vi "FPGA_AIWriteAccumulatorCenter.vi"(8 "error in (no error)":errorcluster, 9 "Center":i32, 10 "Channel":T1=enum."AI 1", 11 "AI Reference in":T2) -> (0 "error out":errorcluster, 3 "AI Reference out":T2)   [LabVIEW 2017]
uses:
  <vilib>/Rock Robotics/SystemInterfaces/AI/FPGA_AIDevRef.ctl
  <vilib>/Rock Robotics/SystemInterfaces/AI/FPGA_AIChannel.ctl
  <vilib>/Rock Robotics/SystemInterfaces/System/FPGA_SystemFPGA Ref Global.vi
  <vilib>/Utility/error.llb/Error Cluster From Error Code.vi
  <vilib>/rvi/errors/niLvFpgaAdjustHostInterfaceError.vi
  <vilib>/rvi/interface/nirviReadWriteControl/nirviReadWriteControl.xnode
  <vilib>/Rock Robotics/SystemInterfaces/System/FPGA_SystemFRC FPGA Ref.ctl
  <vilib>/rvi/interface/Simulation/niFpgaSimulationCallBeginRW.vi
  NiFpgaLv.dll
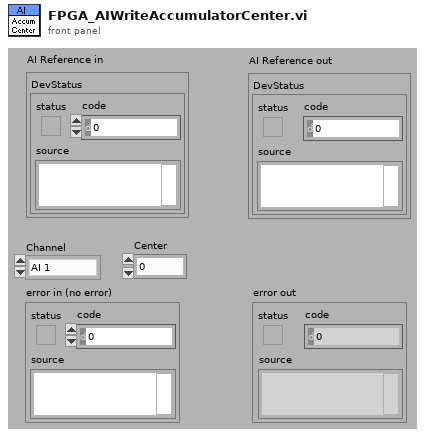
[diagram p1: front panel]
types:
  T1 = typedef "FPGA_AIChannel.ctl" = enum8{"AI 0", "AI 1", "AI 2", "AI 3", "AI MXP 0", "AI MXP 1", "AI MXP 2", "AI MXP 3", "Invalid"}
  T2 = typedef "FPGA_AIDevRef.ctl" = cluster{"DevStatus":errorcluster}
  T3 = typedef "FPGA_SystemFRC FPGA Ref.ctl" = refnum<k20>
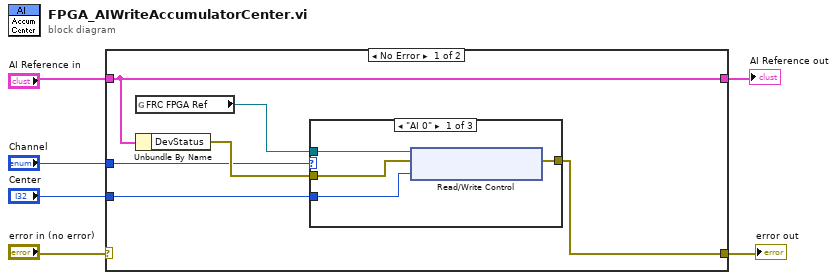
[diagram p0: block diagram]
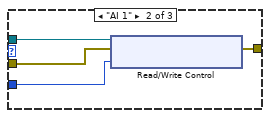
[diagram p2: hidden frame]
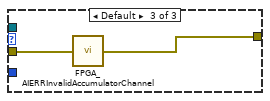
[diagram p3: hidden frame]
diagram:
  n1 = case shown="No Error" "error in (no error)" {
    selector: "error in (no error)" -> [_ w23]
    tunnel: [w12 w24] -> w5
    tunnel: "AI Reference in" -> [w12 w24]
    tunnel: [w9 w23] -> w3
    tunnel: "Center" -> [w10 _]
    tunnel: "Channel" -> [w8 _]
    frame No Error {
      n2 = global read "FPGA_SystemFPGA Ref Global.vi" "FRC FPGA Ref"() -> (w7:T3)
      n3 = Unbundle By Name(w12) -> ("DevStatus"=w11:errorcluster)
      n4 = case shown="\"AI 0\"" w8 {
        tunnel: w11 -> [w14 w18 w22]
        tunnel: [w16 w19 w21] -> w9
        tunnel: w10 -> [w15 w20 _]
        tunnel: w7 -> [w13 w17 _]
        frame "AI 0" {
          n5 = xnode "Read/Write Control"("FPGA VI Reference In"=w13, "error in"=w14, "Accumulator0.Center"=w15) -> ("error out"=w16:errorcluster)  [unwired: 1 out]
        }
        frame "AI 1" {
          n6 = xnode "Read/Write Control"("FPGA VI Reference In"=w17, "error in"=w18, "Accumulator1.Center"=w20) -> ("error out"=w19:errorcluster)  [unwired: 1 out]
        }
        frame Default {
          n7 = call <vilib>:"FPGA_AIERRInvalidAccumulatorChannel.vi"("error in (no error)"=w22) -> ("error out"=w21:errorcluster)
        }
      }
    }
    frame Error {
    }
  }
  "AI Reference out" <- w5
  "error out" <- w3
